vi "System Shutdown.vi"(8 "error in (no error)":errorcluster, 11 "Application in":refnum<class "Application.lvclass">) -> (0 "error out":errorcluster, 3 "Application out":refnum<class "Application.lvclass">)   [LabVIEW 2019, in "Application.lvclass"]
doc: "Developed by Kevin Thompson\nkevin@thompsonengineering.net\n\nCopyright 2018\nThompson Engineering, LLC"
uses:
  Application.lvclass
  Application.lvclass/Application.ctl
  Subsystems/Config/Config.lvclass/Config.ctl
  Accessors/Get Settings.vi
  Subsystems/Config/Accessors/Set Application Settings.vi
  Subsystems/Config/Config.lvclass
  Subsystems/Main/Main.lvclass
  Common/ErrorHandler/ErrorHandler.lvclass
  Subsystems/DAQ_Engine/DAQ_Engine.lvclass
  Subsystems/Log_Engine/Log_Engine.lvclass
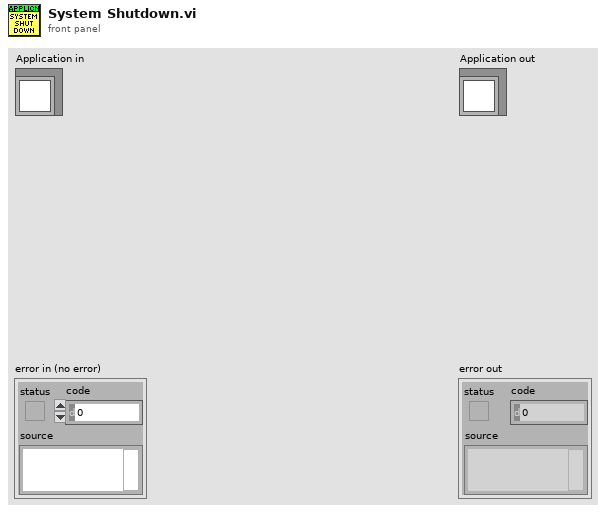
[diagram p1: front panel]
types:
  T1 = typedef "Application.lvclass/Dependency--cluster.ctl" = cluster{"Config":refnum<class "Config.lvclass">, "Main":refnum<class "Main.lvclass">, "ErrorHandler":refnum<class "ErrorHandler.lvclass">, "DAQ_Engine":refnum<class "DAQ_Engine.lvclass">, "Log_Engine":refnum<class "Log_Engine.lvclass">}
  T2 = typedef "Application.lvclass/Settings--cluster.ctl" = cluster{"Simulation":bool}
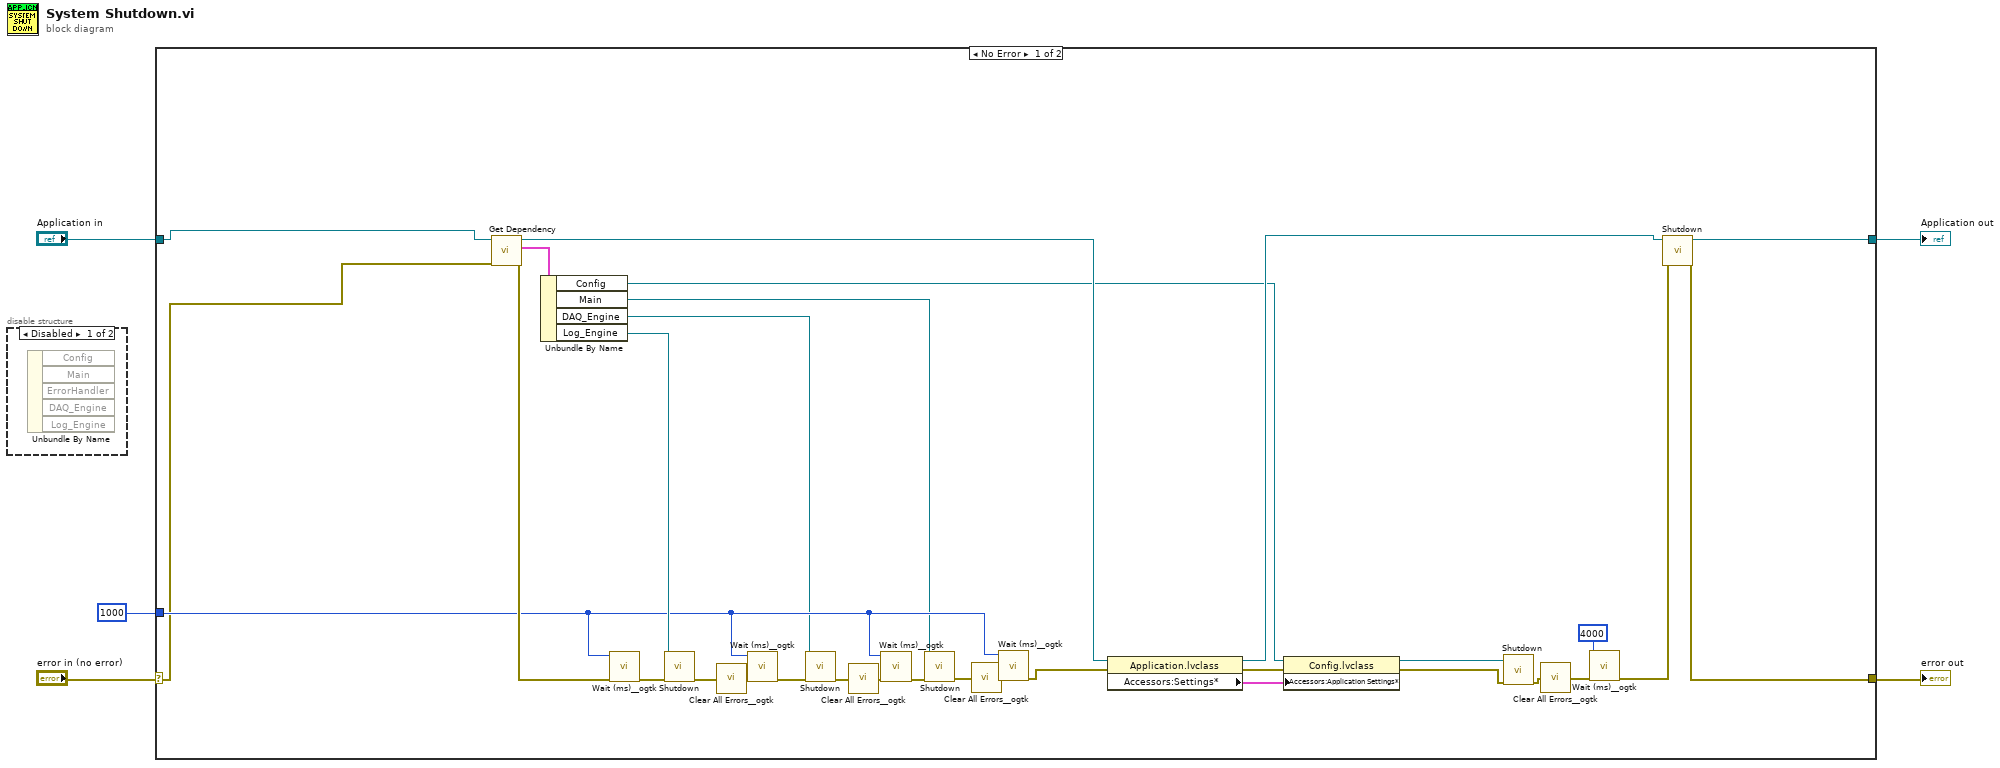
[diagram p0: block diagram]
diagram:
  n1 = disable-structure shown="Disabled" {
    frame Disabled {
      n2 = Unbundle By Name() -> ()  [unwired: 1 in, 5 out]
    }
    frame Enabled {
    }
  }
  n3 = case shown="No Error" "error in (no error)" {
    selector: "error in (no error)" -> [w13 w38]
    tunnel: [w18 w38] -> w4
    tunnel: [w36 w37] -> w2
    tunnel: "Application in" -> [w14 w37]
    tunnel: u32 1000 ("milliseconds to wait") -> [w26 _]
    frame No Error {
      n4 = call "Get Dependency.vi"("error in (no error)"=w13, "Application in"=w14) -> ("error out"=w28:errorcluster, "Dependency"=w35:T1, "Application out"=w12:refnum<class "Application.lvclass">)  [unwired: 7 in]
      n5 = Unbundle By Name(w35) -> ("Config"=w6:refnum<class "Config.lvclass">, "Main"=w17:refnum<class "Main.lvclass">, "DAQ_Engine"=w16:refnum<class "DAQ_Engine.lvclass">, "Log_Engine"=w34:refnum<class "Log_Engine.lvclass">)
      n6 = call <userlib>:"Wait (ms)__ogtk.vi"("error in (no error)"=w28, "milliseconds to wait"=w26) -> ("error out"=w27:errorcluster)  [unwired: 8 in, 1 out]
      n7 = call "Shutdown.vi"("error in (no error)"=w27, "Log_Engine in"=w34) -> ("error out"=w33:errorcluster)  [unwired: 8 in, 1 out]
      n8 = call <userlib>:"Clear All Errors__ogtk.vi"("Error In"=w33) -> ("Error Out"=w23:errorcluster)  [unwired: 3 in]
      n9 = call <userlib>:"Wait (ms)__ogtk.vi"("error in (no error)"=w23, "milliseconds to wait"=w26) -> ("error out"=w32:errorcluster)  [unwired: 8 in, 1 out]
      n10 = call "Shutdown.vi"("error in (no error)"=w32, "DAQ_Engine in"=w16) -> ("error out"=w31:errorcluster)  [unwired: 8 in, 1 out]
      n11 = call <userlib>:"Clear All Errors__ogtk.vi"("Error In"=w31) -> ("Error Out"=w22:errorcluster)  [unwired: 3 in]
      n12 = call <userlib>:"Wait (ms)__ogtk.vi"("error in (no error)"=w22, "milliseconds to wait"=w26) -> ("error out"=w30:errorcluster)  [unwired: 8 in, 1 out]
      n13 = call "Shutdown.vi"("error in (no error)"=w30, "Main in"=w17) -> ("error out"=w29:errorcluster)  [unwired: 8 in, 1 out]
      n14 = call <userlib>:"Clear All Errors__ogtk.vi"("Error In"=w29) -> ("Error Out"=w21:errorcluster)  [unwired: 3 in]
      n15 = call <userlib>:"Wait (ms)__ogtk.vi"("error in (no error)"=w21, "milliseconds to wait"=w26) -> ("error out"=w10:errorcluster)  [unwired: 8 in, 1 out]
      n16 = property class="Application.lvclass"(reference=w12, error in=w10) -> (reference out=w7:refnum<class "Application.lvclass">, error out=w11:errorcluster, "Accessors:Settings*"=w15:T2)
      n17 = property class="Config.lvclass"(reference=w6, error in=w11, "Accessors:Application Settings*"=w15) -> (reference out=w9:refnum<class "Config.lvclass">, error out=w8:errorcluster)
      n18 = call "Shutdown.vi"("error in (no error)"=w8, "Config in"=w9) -> ("error out"=w25:errorcluster)  [unwired: 8 in, 1 out]
      n19 = call <userlib>:"Clear All Errors__ogtk.vi"("Error In"=w25) -> ("Error Out"=w20:errorcluster)  [unwired: 3 in]
      n20 = call <userlib>:"Wait (ms)__ogtk.vi"("error in (no error)"=w20, "milliseconds to wait"=u32 4000) -> ("error out"=w19:errorcluster)  [unwired: 8 in, 1 out]
      n21 = call "Shutdown.vi"("error in (no error)"=w19, "Application in"=w7) -> ("error out"=w18:errorcluster, "Application out"=w36:refnum<class "Application.lvclass">)  [unwired: 8 in]
    }
    frame Error {
    }
  }
  "error out" <- w4
  "Application out" <- w2
